vi "test18-LosslessRegisterStateMultipleTimesNonCSM.vi"(8 "error in (no error)":errorcluster, 11 "TestCase in":refnum<class "testcase-CSMBroadcast.lvclass">) -> (0 "error out":errorcluster, 3 "TestCase out":refnum<class "testcase-CSMBroadcast.lvclass">)   [LabVIEW 2017, in "testcase-CSMBroadcast.lvclass"]
uses:
  testcase-CSMBroadcast.lvclass
  <vilib>/addons/_JKI Toolkits/VI Tester/TestCase.llb/TestCase.lvclass
  src/user.lib/_NEVSTOP/Communicable State Machine(CSM)/Communicable State Machine.lvlib
  CSM/CSM-Testcase.lvlib
  C:/Program Files (x86)/National Instruments/LabVIEW 2017/vi.lib/addons/_JKI Toolkits/VI Tester/TestCase.llb/TestCase.lvclass
panel:
  out "Arguments":string
  out "ModuleName":string
  out "LoopCount":i32
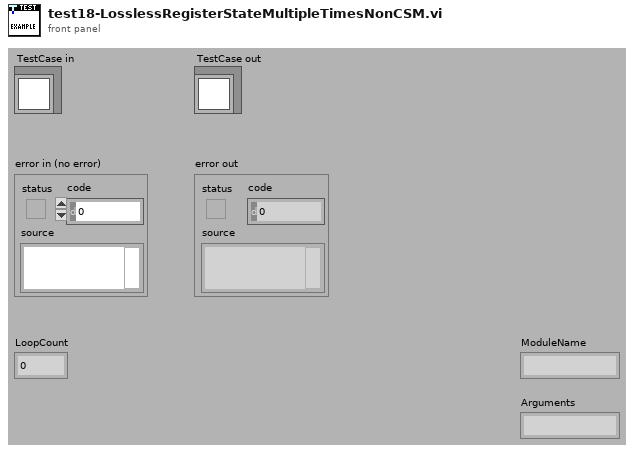
[diagram p1: front panel]
types:
  T1 = cluster{"ModuleName":string, "Status":string, "Arguments":string}
  T2 = cluster{"cluster":cluster{"ModuleName":string, "Status":string, "Arguments":string}, "Counter":u32}
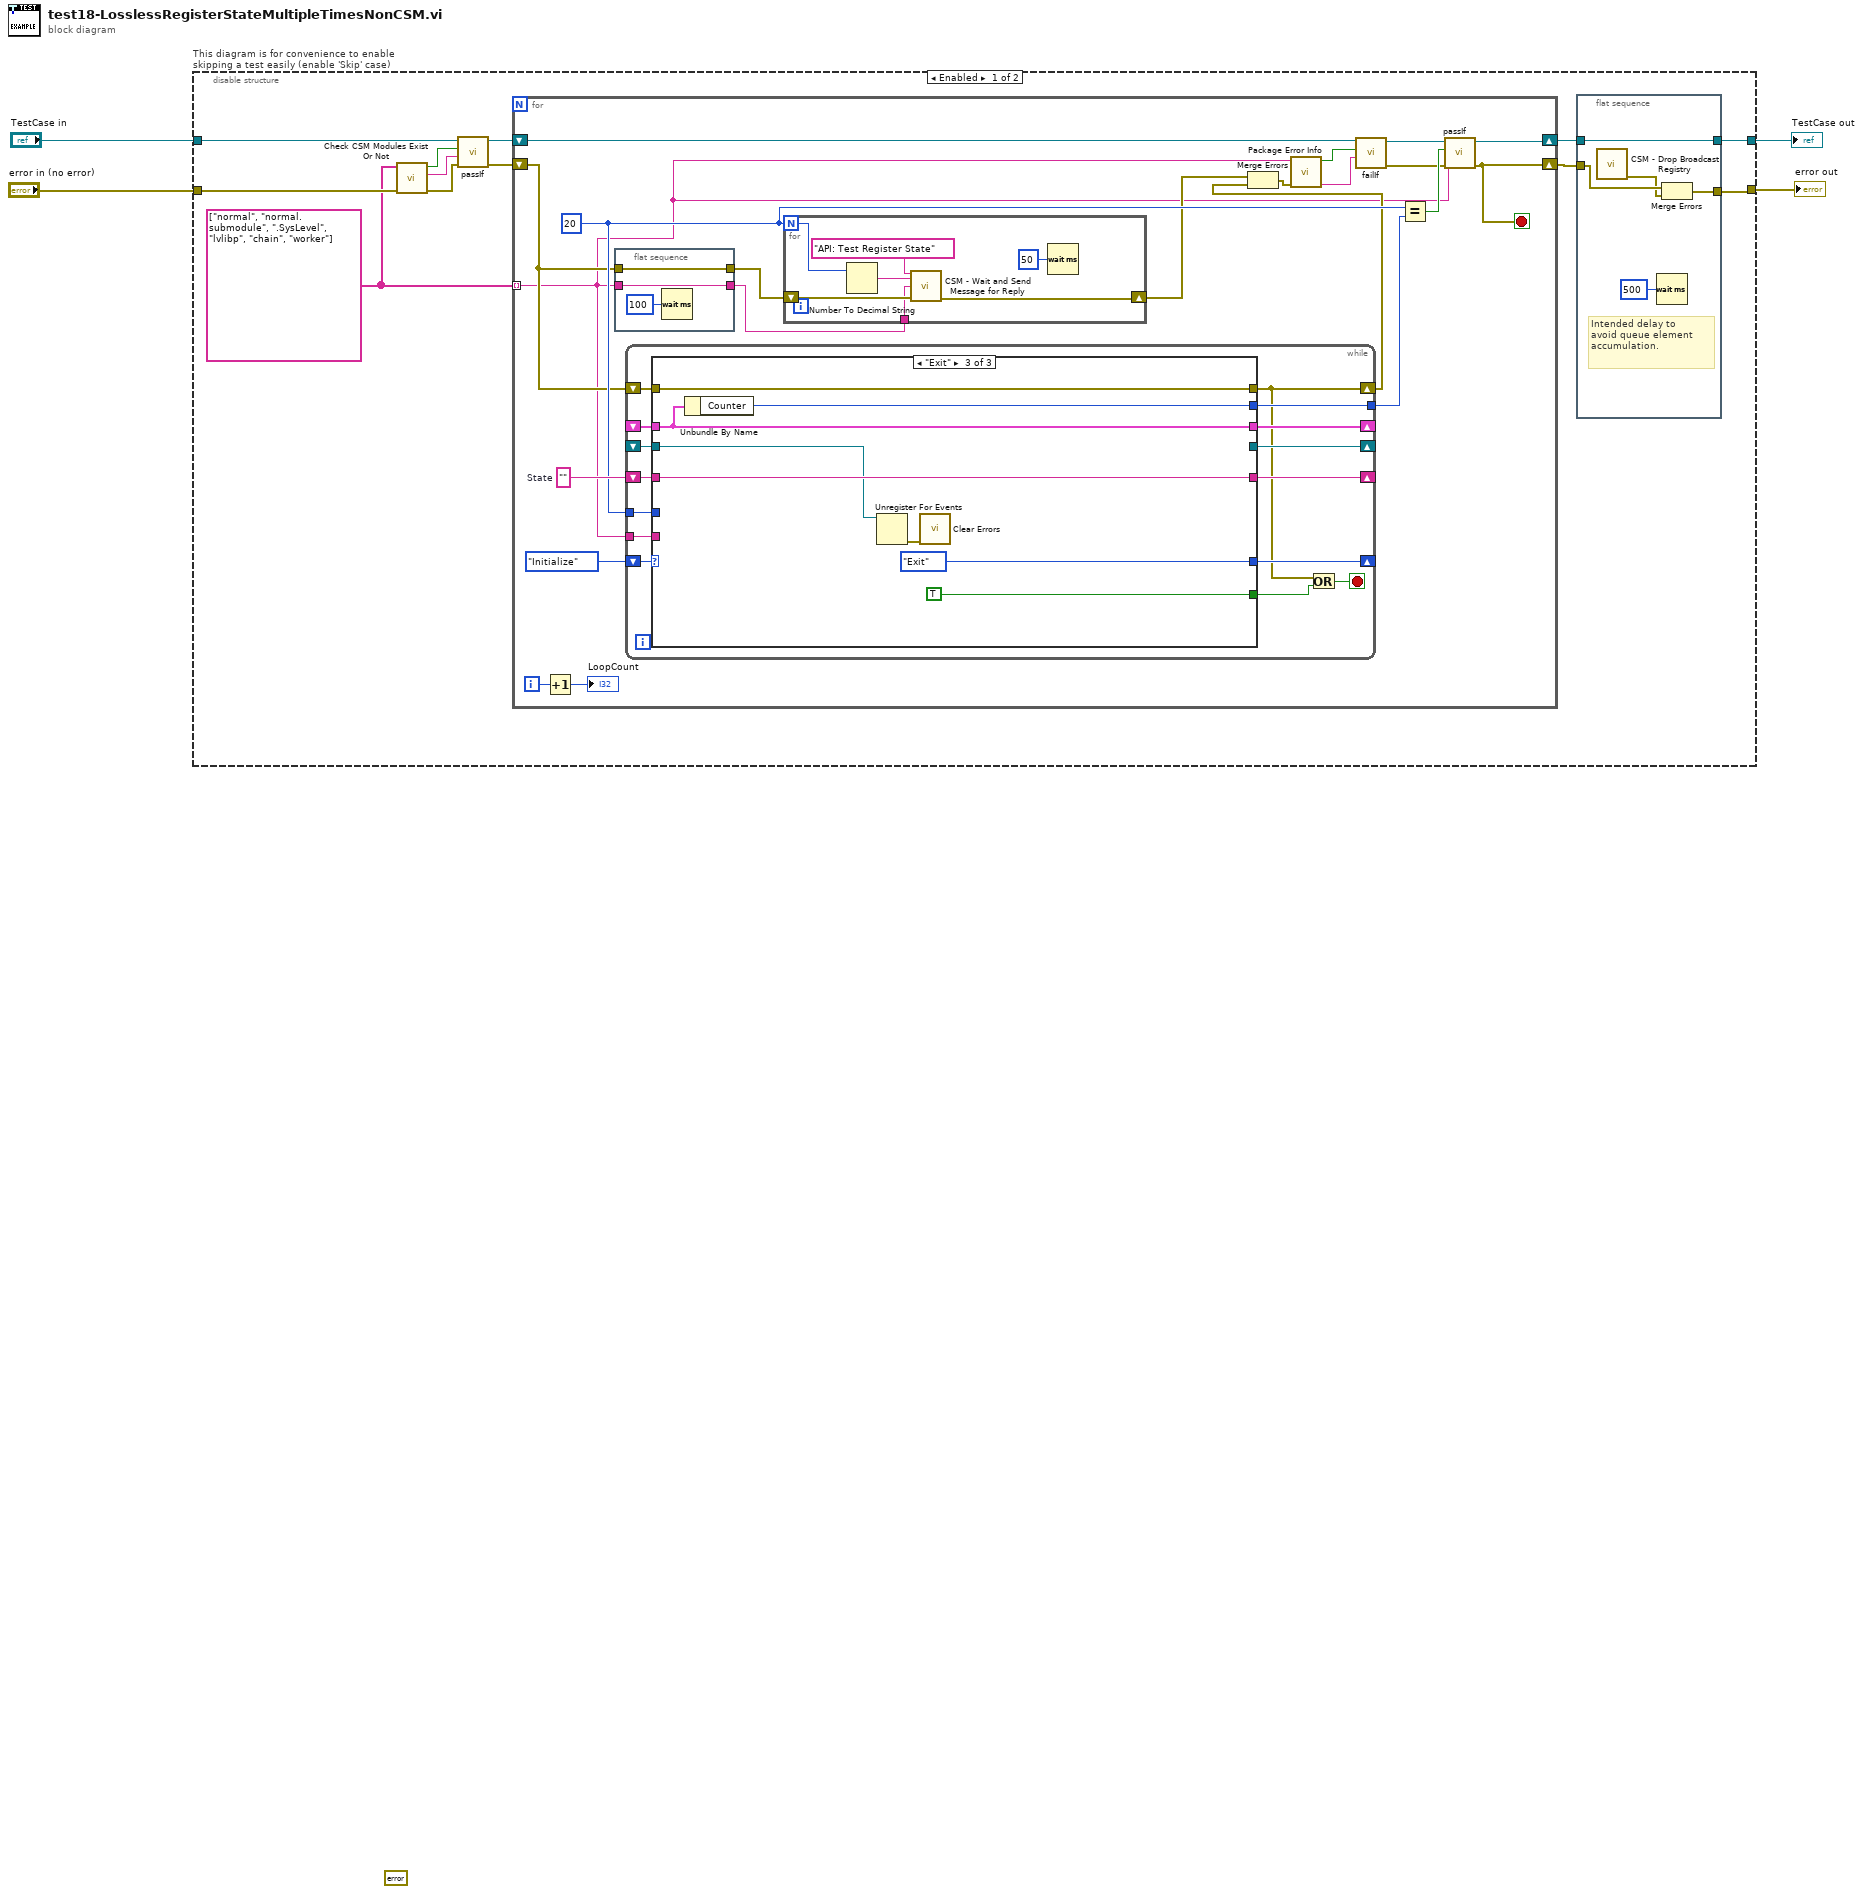
[diagram p0: block diagram]
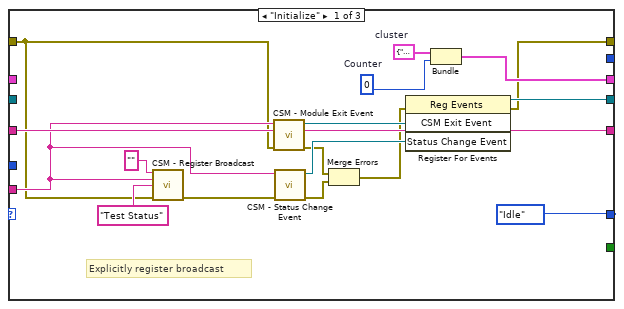
[diagram p2: hidden frame]
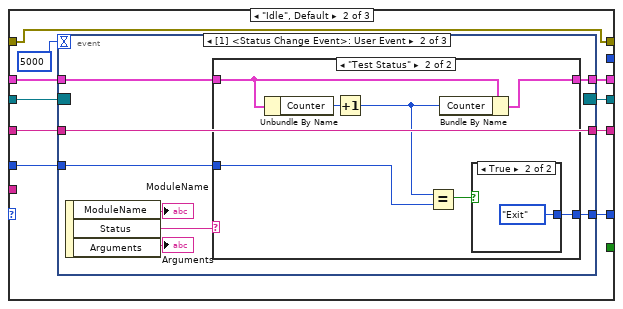
[diagram p3: hidden frame]
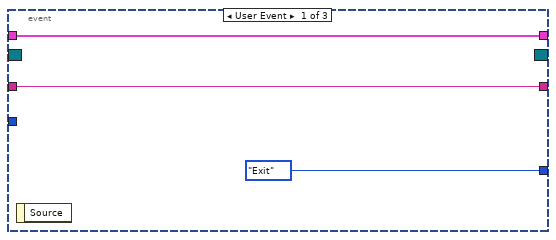
[diagram p4: hidden frame]
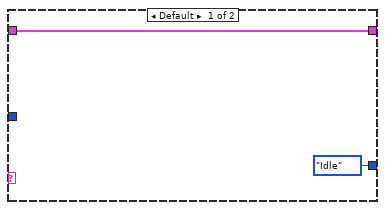
[diagram p5: hidden frame]
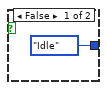
[diagram p6: hidden frame]
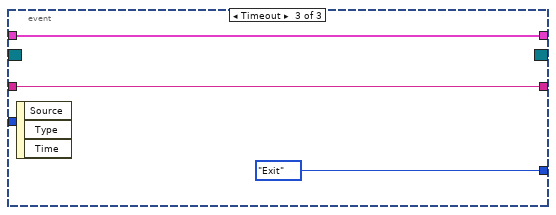
[diagram p7: hidden frame]
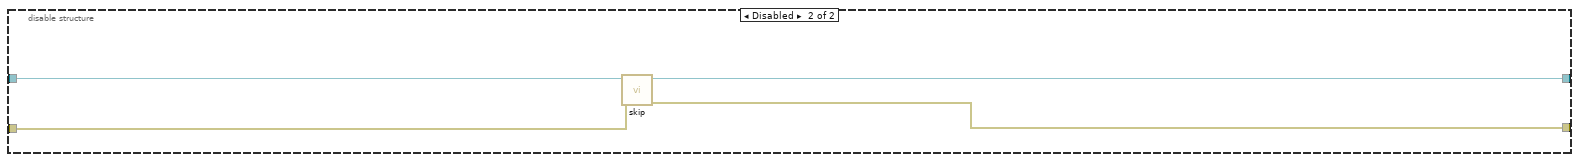
[diagram p8: hidden frame]
diagram:
  (unwired) errorcluster {"status"=FALSE, "code"=0, "source"=""} ("error out")
  n1 = disable-structure "This diagram is for convenience to enable skipping a test easily (enable 'Skip' case)" shown="Enabled" {
    disable-tunnel: "TestCase in" -> [w11 w131]
    disable-tunnel: [w5 w129] -> w2
    disable-tunnel: [w15 w130] -> w1
    disable-tunnel: "error in (no error)" -> [w8 w128]
    frame Enabled {
      w7 = string[] ["normal", "normal.submodule", ".SysLevel", "lvlibp", "chain", "worker"]
      n2 = call "Check CSM Modules Exist Or Not.vi"("error in"=w8, "CSM names in"=w7) -> ("error out"=w12:errorcluster, "Debug string"=w13:string, "All Modules Exist?"=w14:bool)  [unwired: 7 in]
      n3 = call-dynamic "passIf.vi"("error in (no error)"=w12, "message (\"\")"=w13, "pass"=w14, "TestCase in"=w11) -> ("error out"=w9:errorcluster, "TestCase out"=w10:refnum<class "testcase-CSMBroadcast.lvclass">)  [unwired: 6 in]
      n4 = for {
        shift-right: [w40] -> w6
        shift-left: w10 -> [w24]
        shift-right: [w37] -> w16
        shift-left: w9 -> [w31]
        tunnel: w7 -> [w25] mode=indexing
        i -> [w39]
        stop <- w37 stop-if-true
        w33 = 20
        w41 = ""  # State
        n5 = Increment(x=w39) -> (x+1=→"LoopCount":i32)
        n6 = flat-sequence {
          tunnel: w25 -> [w52]
          tunnel: [w52] -> w36
          tunnel: w31 -> [w50]
          tunnel: [w50] -> w32
          frame #0 {
            n7 = Wait (ms)(milliseconds to wait=u32 100) -> ()  [unwired: 1 out]
          }
        }
        n8 = while {
          shift-right: [w66] -> _
          shift-left: enum16{"Idle", "Initialize", "Exit"}."Initialize" -> [w67]
          shift-right: [w64] -> _
          shift-left: w41 -> [w65]
          shift-right: [w63] -> _
          shift-left: _ -> [w62]
          shift-right: [w61] -> _
          shift-left: _ -> [w60]
          tunnel: w25 -> [w59]
          tunnel: [w58] -> w35
          tunnel: w33 -> [w57]
          shift-right: [w55] -> w28
          shift-left: w31 -> [w56]
          stop <- w53 stop-if-true
          n9 = case shown="\"Exit\"" w67 {
            tunnel: [enum16{"Idle", "Initialize", "Exit"}."Idle" w94 enum16{"Idle", "Initialize", "Exit"}."Exit"] -> w66
            tunnel: [_ _ TRUE] -> w54
            tunnel: w65 -> [w83 w92 w125]
            tunnel: [w83 w93 w125] -> w64
            tunnel: [w81 w90 _] -> w63
            tunnel: w62 -> [_ w91 w124]
            tunnel: [w80 w88 w121] -> w61
            tunnel: w60 -> [_ w89 w121]
            tunnel: w59 -> [w72 _ _]
            tunnel: [_ _ w122] -> w58
            tunnel: w57 -> [_ w86 _]
            tunnel: w56 -> [w70 w85 w120]
            tunnel: [w68 w85 w120] -> w55
            frame "Initialize" {
              w75 = u32 0  # Counter
              w78 = T1 {"ModuleName"="", "Status"="", "Arguments"=""}  # cluster
              # "Explicitly register broadcast"
              n10 = call "CSM - Register Broadcast.vi"("CSM Name(Empty for Broadcast Event)"="", "Source CSM Name (* as Default)"=w72, "Trigger"="Test Status" ("State"), "Error In"=w70) -> ("error out"=w71:errorcluster)  [unwired: 10 in, 1 out]
              n11 = call "CSM - Module Exit Event.vi"("Error In"=w70, "Name (\"\" to Use UUID) In"=w72) -> ("error out"=w77:errorcluster, "CSM Exit Event"=w82:refnum<user-event>)  [unwired: 7 in, 1 out]
              n12 = call "CSM - Status Change Event.vi"("Error In"=w71, "CSM Module"=w72) -> ("error out"=w76:errorcluster, "Status Change Event"=w79:refnum<user-event>)  [unwired: 7 in, 1 out]
              n13 = Merge Errors(w77, w76) -> (w69:errorcluster)
              n14 = register-events(error in=w69, w82, w79) -> (reference out=w81:refnum<event-registration>, error out=w68:errorcluster)  [unwired: 1 in]
              n15 = Bundle("cluster"=w78, "Counter"=w75) -> (w80:T2)  [unwired: 1 in]
            }
            frame "Idle", Default {
              n16 = event shown="[1] <Status Change Event>: User Event" {
                selector: w91 -> [_ _ _]
                dyn-events: [_ _ _] -> w90
                timeout: 5000 -> [_ _ _]
                tunnel: [enum16{"Idle", "Initialize", "Exit"}."Exit" w104 enum16{"Idle", "Initialize", "Exit"}."Exit"] -> w94
                tunnel: w92 -> [w97 w105 w119]
                tunnel: [w97 w105 w119] -> w93
                tunnel: w89 -> [w95 w102 w118]
                tunnel: [w95 w103 w118] -> w88
                tunnel: w86 -> [_ w101 _]
                event User Event {
                  n17 = event-data() -> ()  [unwired: 1 in, 1 out]
                }
                event User Event {
                  n18 = event-data() -> ("ModuleName"=→"ModuleName":string, "Status"=w100:string, "Arguments"=→"Arguments":string)  [unwired: 1 in]
                  n19 = case shown="\"Test Status\"" w100 {
                    tunnel: [enum16{"Idle", "Initialize", "Exit"}."Idle" w114] -> w104
                    tunnel: [w107 w113] -> w103
                    tunnel: w102 -> [w107 w112]
                    tunnel: w101 -> [_ w108]
                    frame Default {
                    }
                    frame "Test Status" {
                      n20 = Unbundle By Name(w112) -> ("Counter"=w111:u32)
                      n21 = Increment(x=w111) -> (x+1=w109:u32)
                      n22 = Equal?(x=w109, y=w108) -> (x = y?=w110:bool)
                      n23 = Bundle By Name(cluster=w112, "Counter"=w109) -> (w113:T2)
                      n24 = case shown="True" w110 {
                        tunnel: [enum16{"Idle", "Initialize", "Exit"}."Idle" enum16{"Idle", "Initialize", "Exit"}."Exit"] -> w114
                        frame False {
                        }
                        frame True {
                        }
                      }
                    }
                  }
                }
                event Timeout {
                  n25 = event-data() -> ()  [unwired: 1 in, 3 out]
                }
              }
            }
            frame "Exit" {
              n26 = Unbundle By Name(w121) -> ("Counter"=w122:u32)
              n27 = Unregister For Events(event registration refnum=w124) -> (error out=w123:errorcluster)  [unwired: 1 in]
              n28 = call <vilib>:"Clear Errors.vi"("error in (no error)"=w123) -> ()  [unwired: 5 in, 2 out]
            }
          }
          n29 = Or(x=w55, y=w54) -> (x .or. y?=w53:bool)
        }
        n30 = for {
          N: w33 -> [w47]
          shift-right: [w45] -> w26
          shift-left: w32 -> [w46]
          tunnel: w36 -> [w44]
          n31 = Number To Decimal String(number=w47) -> (decimal integer string=w48:string)  [unwired: 1 in]
          n32 = call "CSM - Wait and Send Message for Reply.vi"("State"="API: Test Register State", "Arguments (\"\")"=w48, "Target Module"=w44, "Error In (No Error)"=w46) -> ("error out"=w45:errorcluster)  [unwired: 8 in, 3 out]
          n33 = Wait (ms)(milliseconds to wait=u32 50) -> ()  [unwired: 1 out]
        }
        n34 = Merge Errors(w26, w28) -> (w27:errorcluster)
        n35 = call "Package Error Info.vi"("error in"=w27, "String in"=w25) -> ("packed error info out"=w29:string, "error status"=w30:bool)  [unwired: 8 in]
        n36 = call-dynamic "failIf.vi"("message (\"\")"=w29, "fail"=w30, "TestCase in"=w24) -> ("error out"=w22:errorcluster, "TestCase out"=w23:refnum<class "testcase-CSMBroadcast.lvclass">)  [unwired: 7 in]
        n37 = Equal?(x=w33, y=w35) -> (x = y?=w34:bool)
        n38 = call-dynamic "passIf.vi"("error in (no error)"=w22, "message (\"\")"=w25, "pass"=w34, "TestCase in"=w23) -> ("error out"=w37:errorcluster, "TestCase out"=w40:refnum<class "testcase-CSMBroadcast.lvclass">)  [unwired: 6 in]
      }
      n39 = flat-sequence {
        tunnel: w16 -> [w21]
        tunnel: [w20] -> w15
        tunnel: w6 -> [w18]
        tunnel: [w18] -> w5
        frame #0 {
          # "Intended delay to\navoid queue element\naccumulation."
          n40 = call "CSM - Drop Broadcast Registry.vi"() -> ("error out"=w19:errorcluster)  [unwired: 15 in]
          n41 = Wait (ms)(milliseconds to wait=u32 500) -> ()  [unwired: 1 out]
          n42 = Merge Errors(w21, w19) -> (w20:errorcluster)
        }
      }
    }
    frame Disabled {
      # "skip test result while test is under development"
      n43 = call <vilib>:"skip.vi"("error in (no error)"=w128, "TestCase in"=w131) -> ("error out"=w130:errorcluster, "TestCase out"=w129:refnum<class "testcase-CSMBroadcast.lvclass">)  [unwired: 8 in]
    }
  }
  "error out" <- w1
  "TestCase out" <- w2
